vi "R-T Fit and Plot.vi"() -> ()   [LabVIEW 2017]
panel:
  out "XY Graph 2":cluster{"X":dbl, "Y":dbl}[](graph)
  out "Best-Fit Coefficients":dbl[](array[numeric])
  out "XY Graph":T1(graph)
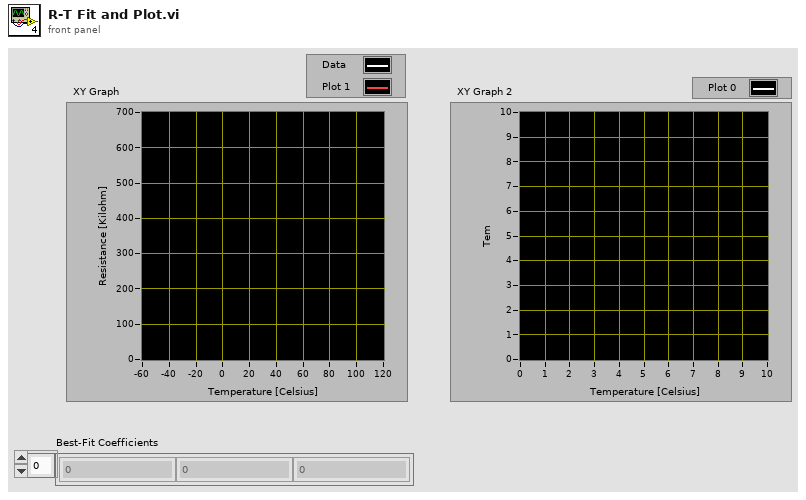
[diagram p1: front panel]
types:
  T1 = cluster{"T [Celsius]":dbl[], "R [kilohm]":dbl[]}[]
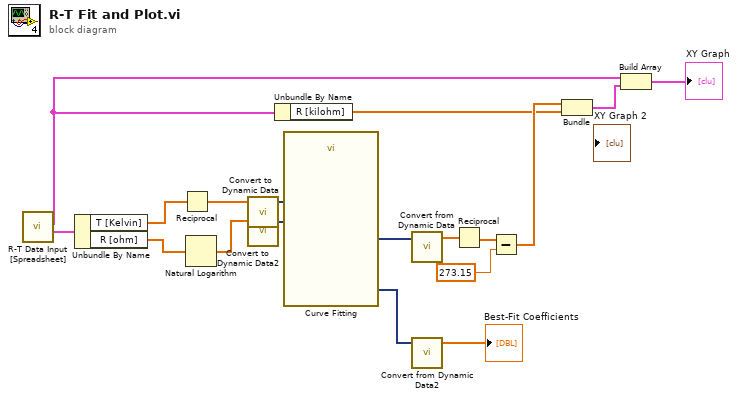
[diagram p0: block diagram]
diagram:
  n1 = call "R-T Data Input [Spreadsheet].vi"() -> ("Kelvin-ohm"=w18:cluster{"T [Kelvin]":dbl[], "R [ohm]":dbl[]}, "Celsius -kilohm"=w4:cluster{"T [Celsius]":dbl[], "R [kilohm]":dbl[]})  [unwired: 10 in]
  n2 = Unbundle By Name(w18) -> ("T [Kelvin]"=w17:dbl[], "R [ohm]"=w16:dbl[])
  n3 = Reciprocal(x=w17) -> (1/x=w15:dbl[])
  n4 = Natural Logarithm(1:w16) -> (0:w13:dbl[])
  n5 = call "Convert to Dynamic Data"("Array"=w15) -> ("Dynamic Data Type"=w14:dynamicdata)  [unwired: 3 in]
  n6 = call "Convert to Dynamic Data2"("Array"=w13) -> ("Dynamic Data Type"=w12:dynamicdata)  [unwired: 3 in]
  n7 = Unbundle By Name(w4) -> ("R [kilohm]"=w5:dbl[])
  n8 = call "Curve Fitting"("Locations"=w12, "Signals"=w14) -> ("best fit"=w11:dynamicdata, "general LS coefficients"=w1:dynamicdata)  [unwired: 5 in, 3 out]
  n9 = call "Convert from Dynamic Data"("Dynamic Data Type"=w11) -> ("Array"=w10:dbl[])  [unwired: 3 in]
  n10 = call "Convert from Dynamic Data2"("Dynamic Data Type"=w1) -> ("Array"=→"Best-Fit Coefficients":dbl[])  [unwired: 3 in]
  n11 = Reciprocal(x=w10) -> (1/x=w9:dbl[])
  n12 = Subtract(x=w9, y=273.15) -> (x-y=w6:dbl[])
  n13 = Bundle(w6, "R [kilohm]"=w5) -> (w3:cluster{dbl[], "R [kilohm]":dbl[]})  [unwired: 1 in]
  n14 = Build Array(w4, w3) -> (→"XY Graph":T1)
